vi "New File Handler.vi"(8 "maximum age [days](None)":dbl=nan, 9 "max file size [MB](50)":dbl=50.0, 10 "formatter (JSON)":refnum<class "Formatter.lvclass">, 11 "log directory (<app dir>/logs)":path) -> (3 "file handler":refnum<class "File Handler.lvclass">)   [LabVIEW 2018, in "GLog.lvlib" / "File Handler.lvclass"]
doc: "Creates a new Handler which writes log records to a file."
uses:
  File Handler.lvclass
  C:/Users/Colin/Documents/software_projects/labview/glog/src/api/extension/formatting_handler_interface/Formatting Handler.lvclass
  extension/formatter_interface/Formatter.lvclass
  File Handler.lvclass/File Handler.ctl
  extension/formatting_handler_interface/Formatting Handler.lvclass/Formatting Handler.ctl
  formatters/JSON_formatter/JSON.lvclass
  C:/Users/Colin/Documents/software_projects/labview/glog/src/api/extension/formatter_interface/Formatter.lvclass
  RolloverTrigger.Size/RolloverTrigger.Size.lvclass
  C:/Users/Colin/Documents/software_projects/labview/glog/src/api/configuration/handlers/file_handler/RolloverTrigger/RolloverTrigger.lvclass
  extension/formatting_handler_interface/Formatting Handler.lvclass
panel:
  # "Connector Pane"
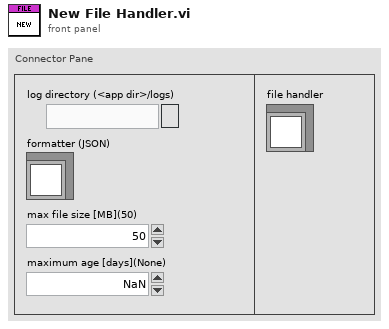
[diagram p1: front panel]
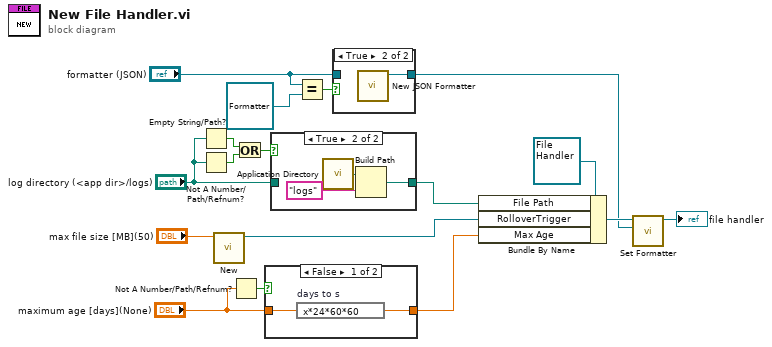
[diagram p0: block diagram]
diagram:
  n1 = Empty String/Path?(string/path="log directory (<app dir>/logs)") -> (empty?=w11:bool)
  n2 = Not A Number/Path/Refnum?(number/path/refnum="log directory (<app dir>/logs)") -> (NaN/Path/Refnum?=w15:bool)
  n3 = call "New.vi"("max file size [MB](50)"="max file size [MB](50)") -> ("size trigger"=w1:refnum<class "RolloverTrigger.Size.lvclass">)  [unwired: 10 in]
  n4 = Not A Number/Path/Refnum?(number/path/refnum="maximum age [days](None)") -> (NaN/Path/Refnum?=w8:bool)
  n5 = Or(x=w11, y=w15) -> (x .or. y?=w12:bool)
  n6 = case shown="False" w8 {
    tunnel: "maximum age [days](None)" -> [w19 w20]
    tunnel: [w18 w20] -> w16
    frame False {
      n7 = expression code="x*24*60*60" "days to s"(w19) -> (w18:dbl)
    }
    frame True {
    }
  }
  n8 = case shown="True" w12 {
    tunnel: "log directory (<app dir>/logs)" -> [w21 _]
    tunnel: [w21 w22] -> w14
    frame False {
    }
    frame True {
      n9 = call <vilib>:"Application Directory.vi"() -> ("Application Directory"=w24:path)
      n10 = Build Path(base path=w24, name or relative path="logs") -> (appended path=w22:path)
    }
  }
  n11 = Equal?(x="formatter (JSON)", y=refnum<class "Formatter.lvclass"> refnum ("formatter (JSON)")) -> (x = y?=w5:bool)
  n12 = case shown="True" w5 {
    tunnel: [w25 w26] -> w6
    tunnel: "formatter (JSON)" -> [w25 _]
    frame False {
    }
    frame True {
      n13 = call "New JSON Formatter.vi"() -> ("JSON formatter"=w26:refnum<class "JSON.lvclass">)  [unwired: 11 in]
    }
  }
  n14 = Bundle By Name(cluster=refnum<class "File Handler.lvclass"> refnum ("file handler"), "File Path"=w14, "RolloverTrigger"=w1, "Max Age"=w16) -> (w10:refnum<class "File Handler.lvclass">)
  n15 = call "Set Formatter.vi"("formatter"=w6, "handler in"=w10) -> ("handler out"=→"file handler":refnum<class "File Handler.lvclass">)  [unwired: 9 in]
